vi "Fonts AE.vi"(7 "Dispose":bool, 8 "error in (no error)":errorcluster, 11 "Font":refnum<class "Font Settings.lvclass">) -> (0 "error out":errorcluster, 3 "Font":refnum<k24>)   [LabVIEW 2023, in "Glyph .NET Drawer.lvlib" / "Drawer .Net.lvclass"]
uses:
  Drawer .Net.lvclass
  Font Glyph Drawer Interface/Font Settings/Font Settings.lvclass
  System.Drawing
  Drawer .Net.lvclass/Drawer .Net.ctl
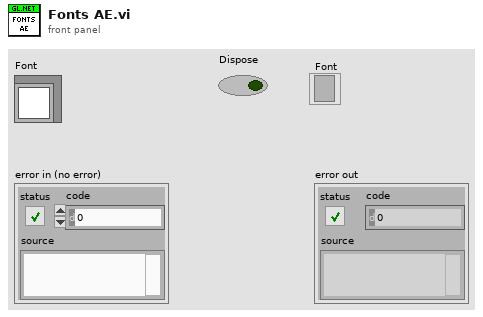
[diagram p1: front panel]
types:
  T1 = map{refnum<class "Font Settings.lvclass">, refnum<k24>}
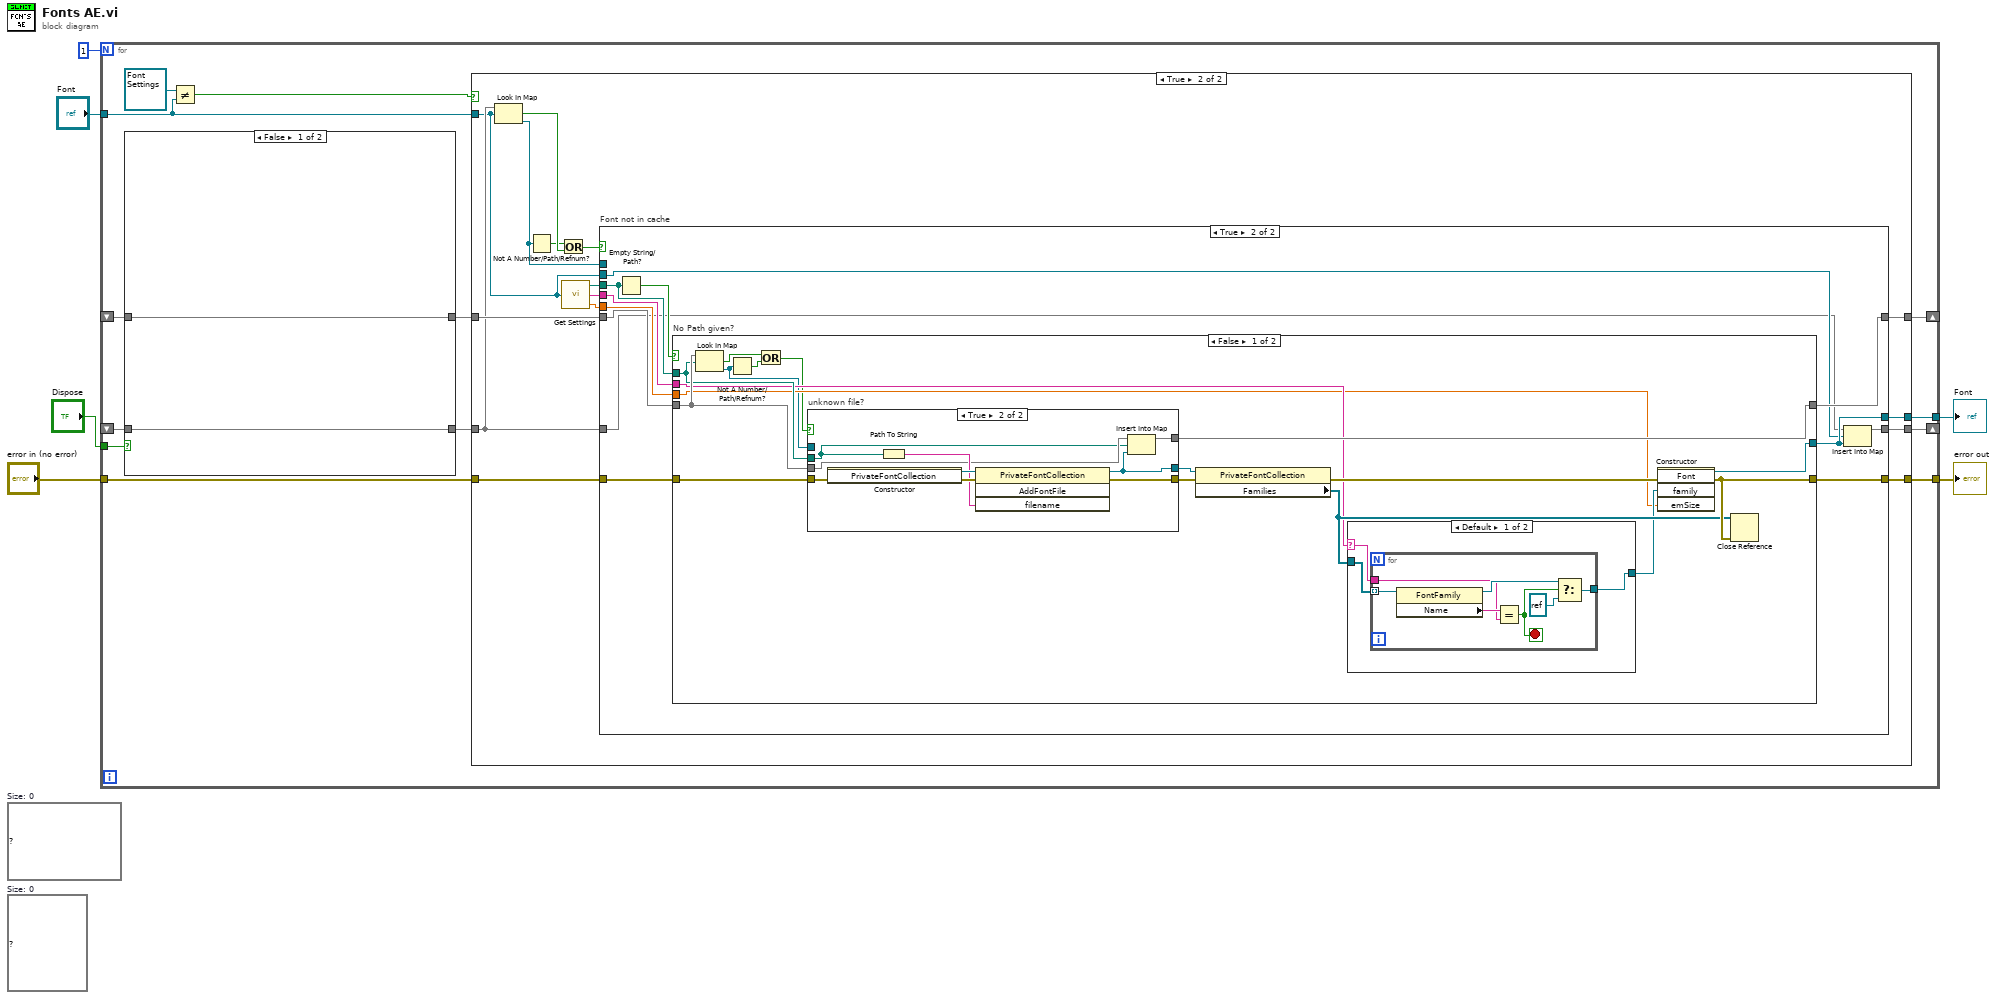
[diagram p0: block diagram]
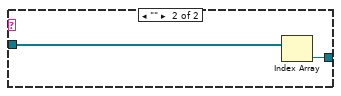
[diagram p4: hidden frame]
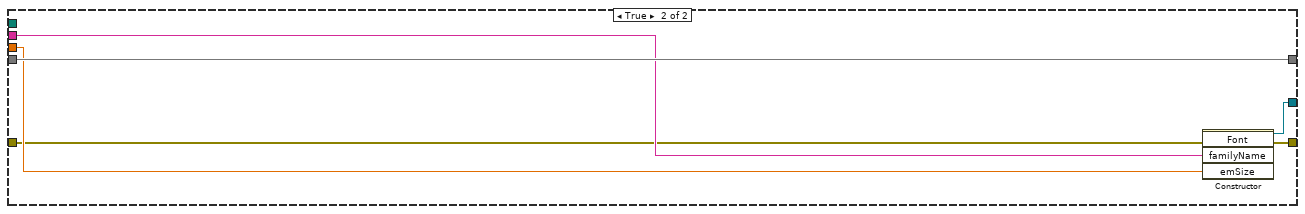
[diagram p6: hidden frame]
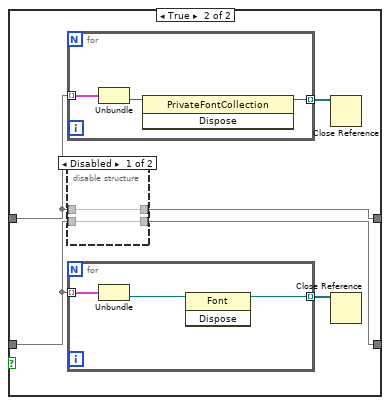
[diagram p7: hidden frame]
diagram:
  (unwired) map{path, refnum<k24>} {}  # Size: 0
  (unwired) T1 {}  # Size: 0
  n1 = for {
    N: 1 -> [_]
    tunnel: "Font" -> [w7]
    shift-right: [w18] -> _
    shift-left: _ -> [w12]
    shift-right: [w19] -> _
    shift-left: _ -> [w13]
    tunnel: [w17] -> w4
    tunnel: "error in (no error)" -> [w16]
    tunnel: [w15] -> w2
    tunnel: "Dispose" -> [w14]
    n2 = case shown="False" w14 {
      tunnel: w13 -> [w102 w106]
      tunnel: w12 -> [w101 w103]
      tunnel: [w102 w107] -> w11
      tunnel: [w101 w104] -> w10
      frame False {
      }
      frame True {
        n3 = for {
          tunnel: w106 -> [w116] mode=indexing
          tunnel: [w114] -> w108 mode=indexing
          n4 = Unbundle(w116) -> ("new reference"=w115:refnum<k24>)  [unwired: 1 out]
          n5 = invoke class="PrivateFontCollection" method="Dispose"(reference=w115) -> (reference out=w114:refnum<k24>)  [unwired: 2 in, 2 out]
        }
        n6 = disable-structure shown="Disabled" {
          disable-tunnel: [w113 _] -> w107
          disable-tunnel: w106 -> [w113 _]
          disable-tunnel: [w112 _] -> w104
          disable-tunnel: w103 -> [w112 _]
          frame Disabled {
          }
          frame Enabled {
          }
        }
        n7 = for {
          tunnel: w103 -> [w111] mode=indexing
          tunnel: [w109] -> w105 mode=indexing
          n8 = Unbundle(w111) -> ("new reference"=w110:refnum<k24>)  [unwired: 1 out]
          n9 = invoke class="Font" method="Dispose"(reference=w110) -> (reference out=w109:refnum<k24>)  [unwired: 2 in, 2 out]
        }
        n10 = Close Reference(reference=w108) -> ()  [unwired: 1 in, 1 out]
        n11 = Close Reference(reference=w105) -> ()  [unwired: 1 in, 1 out]
      }
    }
    n12 = Not Equal?(x=refnum<class "Font Settings.lvclass"> refnum, y=w7) -> (x != y?=w8:bool)
    n13 = case shown="True" w8 {
      tunnel: [w21 w36] -> w19
      tunnel: [w22 w35] -> w18
      tunnel: [_ w34] -> w17
      tunnel: w16 -> [w20 w33]
      tunnel: [w20 w32] -> w15
      tunnel: w11 -> [w21 w29]
      tunnel: w10 -> [w22 w28]
      tunnel: w7 -> [_ w26]
      frame False {
      }
      frame True {
        n14 = Look In Map(map=w28, key=w26) -> (key not found?=w27:bool, value=w25:refnum<k24>)  [unwired: 1 in]
        n15 = Not A Number/Path/Refnum?(number/path/refnum=w25) -> (NaN/Path/Refnum?=w23:bool)
        n16 = Or(x=w23, y=w27) -> (x .or. y?=w24:bool)
        n17 = call "Get Settings.vi"("Font Settings in"=w26) -> ("Font Path"=w37:path, "Font Name"=w31:string, "Size"=w30:dbl)
        n18 = case "Font not in cache" shown="True" w24 {
          tunnel: w37 -> [_ w51]
          tunnel: [w40 w53] -> w36
          tunnel: w29 -> [w40 w52]
          tunnel: [w39 w42] -> w35
          tunnel: w28 -> [w39 w43]
          tunnel: w25 -> [w41 _]
          tunnel: [w41 w45] -> w34
          tunnel: w33 -> [w38 w49]
          tunnel: [w38 w48] -> w32
          tunnel: w26 -> [_ w44]
          tunnel: w31 -> [_ w47]
          tunnel: w30 -> [_ w46]
          frame False {
          }
          frame True {
            n19 = Empty String/Path?(string/path=w51) -> (empty?=w50:bool)
            n20 = case "No Path given?" shown="False" w50 {
              tunnel: w51 -> [w62 _]
              tunnel: [w67 w100] -> w53
              tunnel: w52 -> [w63 w100]
              tunnel: w49 -> [w70 w95]
              tunnel: [w69 w96] -> w48
              tunnel: [w68 w97] -> w45
              tunnel: w47 -> [w58 w99]
              tunnel: w46 -> [w57 w98]
              frame False {
                n21 = Look In Map(map=w63, key=w62) -> (key not found?=w59:bool, value=w56:refnum<k24>)  [unwired: 1 in]
                n22 = Not A Number/Path/Refnum?(number/path/refnum=w56) -> (NaN/Path/Refnum?=w54:bool)
                n23 = Or(x=w59, y=w54) -> (x .or. y?=w55:bool)
                n24 = case "unknown file?" shown="True" w55 {
                  tunnel: w70 -> [w84 w94]
                  tunnel: [w83 w93] -> w67
                  tunnel: [w84 w92] -> w64
                  tunnel: w63 -> [w83 w88]
                  tunnel: w62 -> [_ w87]
                  tunnel: [w85 w86] -> w60
                  tunnel: w56 -> [w85 _]
                  frame False {
                  }
                  frame True {
                    n25 = constructor class="PrivateFontCollection"(error in=w94) -> (reference out=w90:refnum<k24>, error out=w91:errorcluster)  [unwired: 2 in, 1 out]
                    n26 = Path To String(path=w87) -> (string=w89:string)
                    n27 = invoke class="PrivateFontCollection" method="AddFontFile"(reference=w90, error in=w91, "filename"=w89) -> (reference out=w86:refnum<k24>, error out=w92:errorcluster)  [unwired: 1 in, 2 out]
                    n28 = Insert Into Map(map in=w88, key=w87, value=w86) -> (map out=w93:map{path, refnum<k24>})  [unwired: 2 out]
                  }
                }
                n29 = property class="PrivateFontCollection"(reference=w60, error in=w64) -> (error out=w65:errorcluster, "Families"=w66:refnum<k24>[])  [unwired: 1 out]
                n30 = case shown="Default" w58 {
                  selector: w58 -> [w71 _]
                  tunnel: w66 -> [w73 w82]
                  tunnel: [w72 w81] -> w61
                  frame Default {
                    n31 = for {
                      tunnel: w73 -> [w80] mode=indexing
                      tunnel: [w76] -> w72
                      tunnel: w71 -> [w77]
                      stop <- w75 stop-if-true
                      n32 = property class="FontFamily"(reference=w80) -> (reference out=w79:refnum<k24>, "Name"=w78:string)  [unwired: 1 in, 1 out]
                      n33 = Equal?(x=w78, y=w77) -> (x = y?=w75:bool)
                      n34 = Select(t=w79, s=w75, f=refnum<k24> refnum) -> (s? t:f=w76:refnum<k24>)
                    }
                  }
                  frame "" {
                    n35 = Index Array(array=w82) -> (element=w81:refnum<k24>)  [unwired: 1 in]
                  }
                }
                n36 = constructor class="Font"(error in=w65, "family"=w61, "emSize"=w57) -> (reference out=w68:refnum<k24>, error out=w69:errorcluster)  [unwired: 2 in, 3 out]
                n37 = Close Reference(reference=w66, error in (no error)=w69) -> ()  [unwired: 1 out]
              }
              frame True {
                n38 = constructor class="Font"(error in=w95, "familyName"=w99, "emSize"=w98) -> (reference out=w97:refnum<k24>, error out=w96:errorcluster)  [unwired: 2 in, 3 out]
              }
            }
            n39 = Insert Into Map(map in=w43, key=w44, value=w45) -> (map out=w42:T1)  [unwired: 2 out]
          }
        }
      }
    }
  }
  "Font" <- w4
  "error out" <- w2
